vi "Field Draw Robots.vi"(0 "color":enum16{"Azul", "Amarelo"}(ring), 1 "game in":refnum<class "Game.lvclass">=refnum, 3 "Draw Number":bool=TRUE, 4 "Draw Targets?":T2, 5 "Scale":dbl, 7 "Project":T1=enum."VSS", 9 "Offset":cluster{"Width":dbl, "Height":dbl}, 11 "Picture In":picture, 12 "color(black)":u32, 13 "Lado":enum16{"Esquerdo", "Direito"}(ring), 14 "RobotRef":refnum<class "Robot.lvclass">[](array[class])) -> (6 "Scale Out":dbl, 10 "Offset Out":cluster{"Width":dbl, "Height":dbl}, 15 "Picture Out":picture)   [LabVIEW 2022 SP3]
uses:
  DrawTargets.ctl
  Robot_class/Robot.lvclass
  Game_class/Game.lvclass
  Project.ctl
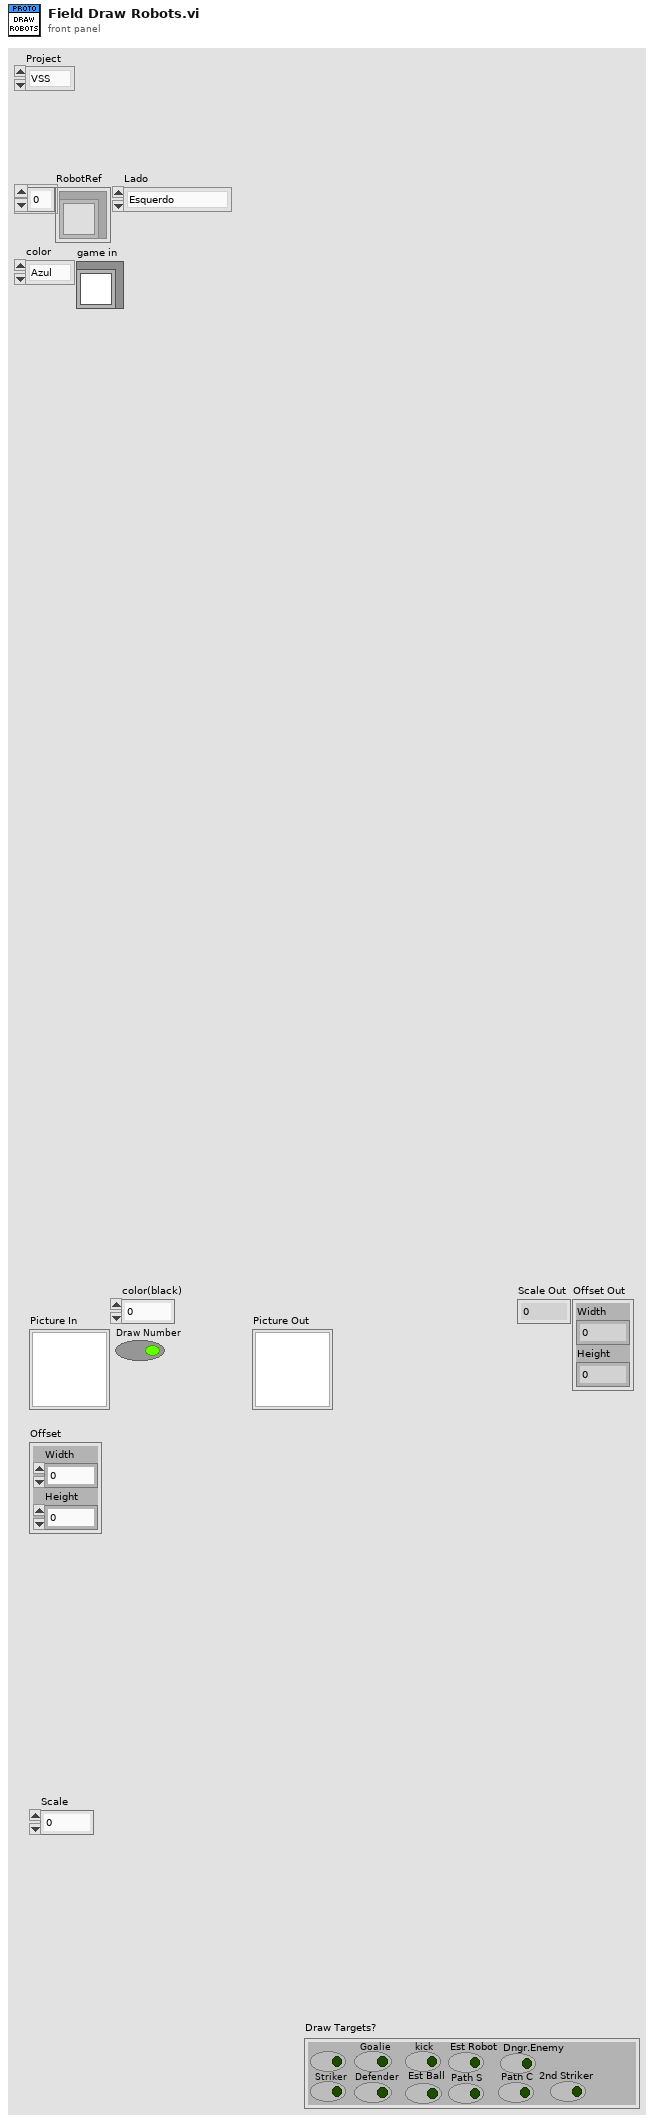
[diagram p1: front panel]
types:
  T1 = typedef "Project.ctl" = enum16{"SSL", "VSS"}
  T2 = typedef "DrawTargets.ctl" = cluster{"Attacker":bool, "Striker":bool, "Goalie":bool, "Defender":bool, "kick":bool, "Est Ball":bool, "Est Robot":bool, "Path S":bool, "Path C":bool, "Dngr.Enemy":bool, "2nd Striker":bool}
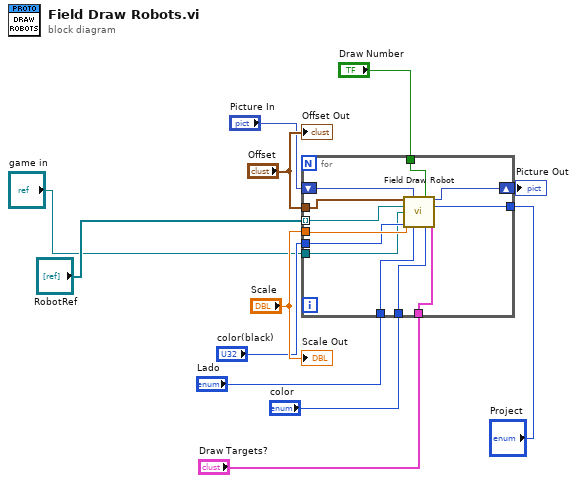
[diagram p0: block diagram]
diagram:
  n1 = for {
    tunnel: "Scale" -> [w20]
    tunnel: "Offset" -> [w21]
    shift-right: [w24] -> w8
    shift-left: "Picture In" -> [w22]
    tunnel: "color(black)" -> [w19]
    tunnel: "Draw Number" -> [w23]
    tunnel: "Draw Targets?" -> [w18]
    tunnel: "RobotRef" -> [w17] mode=indexing
    tunnel: "color" -> [w16]
    tunnel: "Lado" -> [w15]
    tunnel: "game in" -> [w14]
    tunnel: "Project" -> [w13]
    n2 = call "Field Draw Robot.vi"("Offset"=w21, "picture in"=w22, "Draw Number"=w23, "Robot"=w17, "Project"=w13, "Game in"=w14, "Scale mm/pixel"=w20, "color(black)"=w19, "Lado"=w15, "color"=w16, "Draw Targets?"=w18) -> ("picture out"=w24:picture)  [unwired: 4 in]
  }
  "Picture Out" <- w8
  "Scale Out" <- "Scale"
  "Offset Out" <- "Offset"
